vi "Mod_OFDM_Application.vi"(0 "Configure  Modulators Pool":bool, 1 "Configure OFDM Symbol":bool, 2 "Configure OFDM Frame":bool, 3 "Configure Pulse Shaping":bool, 4 "Write Configuration":bool, 5 "error in (no error)":errorcluster, 6 "Configure Data Pool":bool, 7 "Generate Waveform":bool, 8 "Read From File":bool, 9 "EXIT":bool) -> (12 "FFT Spectrum":cluster{dbl, dbl, dbl[]}(graph)={-798437.4999999999, 1562.4999999999998, [-inf, -inf, -inf, -inf, -inf, -inf, -inf, -inf, -inf, -inf, -inf, -inf, -inf, -inf, -inf, -inf, -inf, -inf, -inf, -inf, -inf, -inf, -inf, -inf, -inf, -inf, -inf, -inf, -inf, -inf, -inf, -inf, -inf, -inf, -inf, -inf, -inf, -inf, -inf, -inf, -inf, -inf, -inf, -inf, -inf, -inf, -inf, -inf, -inf, -inf, -inf, -inf, -inf, -inf, -inf, -inf, -inf, -inf, -inf, -inf, -inf, -inf, -inf, -inf, -inf, -inf, -inf, -inf, -inf, -inf, -inf, -inf, -inf, -inf, -inf, -inf, -inf, -inf, -inf, -inf, -inf, -inf, -inf, -inf, -inf, -inf, -inf, -inf, -inf, -inf, -inf, -inf, -inf, -inf, -inf, -inf, -inf, -inf, -inf, -inf, -inf, -inf, -inf, -inf, -inf, -inf, -inf, -inf, -inf, -inf, -inf, -inf, -inf, -inf, -inf, -inf, -inf, -inf, -inf, -inf, -inf, -inf, -inf, -inf, -inf, -inf, -inf, -inf, -inf, -inf, -inf, -inf, -inf, -inf, -inf, -inf, -inf, -inf, -inf, -inf, -inf, -inf, -inf, -inf, -inf, -inf, -inf, -inf, -inf, -inf, -inf, -inf, -inf, -inf, -inf, -inf, -inf, -inf, -inf, -inf, -inf, -inf, -inf, -inf, -inf, -inf, -inf, -inf, -inf, -inf, -inf, -inf, -inf, -inf, -inf, -inf, -inf, -inf, -inf, -inf, -inf, -inf, -inf, -inf, -inf, -inf, -inf, -inf, -inf, -inf, -inf, -inf, -inf, -inf, -inf, -inf, -inf, -inf, -inf, -inf, -inf, -inf, -inf, -inf, -inf, -inf, -inf, -inf, -inf, -inf, -inf, -inf, -inf, -inf, -inf, -inf, -inf, -inf, -inf, -inf, -inf, -inf, -inf, -inf, -inf, -inf, -inf, -inf, -inf, -inf, -inf, -inf, -inf, -inf, -inf, -inf, -inf, -inf, -inf, -inf, -inf, -inf, -inf, -inf, -inf, -inf, -inf, -inf, -inf, -inf, -inf, -inf, -inf, -inf, -inf, -inf, -inf, -inf, -inf, -inf, -inf, -inf, -inf, -inf, -inf, -inf, -inf, -inf, -inf, -inf, -inf, -inf, -inf, -inf, -inf, -inf, -inf, -inf, -inf, -inf, -inf, -inf, -inf, -inf, -inf, -inf, -inf, -inf, -inf, -inf, -inf, -inf, -inf, -inf, -inf, -inf, -inf, -inf, -inf, -inf, -inf, -inf, -inf, -inf, -inf, -inf, -inf, -inf, -inf, -inf, -inf, -inf, -inf, -inf, -inf, -inf, -inf, -inf, -inf, -inf, -inf, -inf, -inf, -inf, -inf, -inf, -inf, -inf, -inf, -inf, -inf, -inf, -inf, -inf, -inf, -inf, -inf, -inf, -inf, -inf, -inf, -inf, -inf, -inf, -inf, -inf, -inf, -inf, -inf, -inf, -inf, -inf, -inf, -inf, -inf, -inf, -inf, -inf, -inf, -inf, -inf, -inf, -inf, -inf, -inf, -inf, -inf, -inf, -inf, -inf, -inf, -inf, -inf, -inf, -inf, -inf, -inf, -inf, -inf, -inf, -inf, -inf, -inf, -inf, -inf, -inf, -inf, -inf, -inf, -inf, -inf, -inf, -inf, -inf, -inf, -inf, -inf, -inf, -inf, -inf, -inf, -inf, -inf, -inf, -inf, -inf, -inf, -inf, -inf, -inf, -inf, -inf, -inf, -inf, -inf, -inf, -inf, -inf, -inf, -inf, -inf, -inf, -inf, -inf, -inf, -inf, -inf, -inf, -inf, -inf, -inf, -inf, -inf, -inf, -inf, -inf, -inf, -inf, -inf, -inf, -inf, -inf, -inf, -inf, -inf, -inf, -inf, -inf, -inf, -inf, -inf, -inf, -inf, -inf, -inf, -inf, -inf, -inf, -inf, -inf, -inf, -inf, -inf, -inf, -inf, -inf, -inf, -inf, -inf, -inf, -inf, -inf, -inf, -inf, -inf, -inf, -inf, -inf, -inf, -inf, -inf, -inf, -inf, -inf, -inf, -inf, -inf, -inf, -inf, -inf, -inf, -inf, -inf, -inf, -inf, -inf, -inf, -inf, -inf, -inf, -inf, -inf, -inf, -inf, -inf, -inf, -inf, -inf, -inf, -inf, -inf, -inf, -inf, -inf, -inf, -inf, -inf, -inf, -inf, -inf, -inf, -inf, -inf, -inf, -inf, -inf, -inf, -inf, -inf, -inf, -inf, -inf, -inf, -inf, -inf, -inf, -inf, -inf, -inf, -inf, -inf, -inf, -inf, -inf, -inf, -inf, -inf, -inf, -inf, -inf, -inf, -inf, -inf, -inf, -inf, -inf, -inf, -inf, -inf, -inf, -inf, -inf, -inf, -inf, -inf, -inf, -inf, -inf, -inf, -inf, -inf, -inf, -inf, -inf, -inf, -inf, -inf, -inf, -inf, -inf, -inf, -inf, -inf, -inf, -inf, -inf, -inf, -inf, -inf, -inf, -inf, -inf, -inf, -inf, -inf, -inf, -inf, -inf, -inf, -inf, -inf, -inf, -inf, -inf, -inf, -inf, -inf, -inf, -inf, -inf, -inf, -inf, -inf, -inf, -inf, -inf, -inf, -inf, -inf, -inf, -inf, -inf, -inf, -inf, -inf, -inf, -inf, -inf, -inf, -inf, -inf, -inf, -inf, -inf, -inf, -inf, -inf, -inf, -inf, -inf, -inf, -inf, -inf, -inf, -inf, -inf, -inf, -inf, -inf, -inf, -inf, -inf, -inf, -inf, -inf, -inf, -inf, -inf, -inf, -inf, -inf, -inf, -inf, -inf, -inf, -inf, -inf, -inf, -inf, -inf, -inf, -inf, -inf, -inf, -inf, -inf, -inf, -inf, -inf, -inf, -inf, -inf, -inf, -inf, -inf, -inf, -inf, -inf, -inf, -inf, -inf, -inf, -inf, -inf, -inf, -inf, -inf, -inf, -inf, -inf, -inf, -inf, -inf, -inf, -inf, -inf, -inf, -inf, -inf, -inf, -inf, -inf, -inf, -inf, -inf, -inf, -inf, -inf, -inf, -inf, -inf, -inf, -inf, -inf, -inf, -inf, -inf, -inf, -inf, -inf, -inf, -inf, -inf, -inf, -inf, -inf, -inf, -inf, -inf, -inf, -inf, -inf, -inf, -inf, -inf, -inf, -inf, -inf, -inf, -inf, -inf, -inf, -inf, -inf, -inf, -inf, -inf, -inf, -inf, -inf, -inf, -inf, -inf, -inf, -inf, -inf, -inf, -inf, -inf, -inf, -inf, -inf, -inf, -inf, -inf, -inf, -inf, -inf, -inf, -inf, -inf, -inf, -inf, -inf, -inf, -inf, -inf, -inf, -inf, -inf, -inf, -inf, -inf, -inf, -inf, -inf, -inf, -inf, -inf, -inf, -inf, -inf, -inf, -inf, -inf, -inf, -inf, -inf, -inf, -inf, -inf, -inf, -inf, -inf, -inf, -inf, -inf, -inf, -inf, -inf, -inf, -inf, -inf, -inf, -inf, -inf, -inf, -inf, -inf, -inf, -inf, -inf, -inf, -inf, -inf, -inf, -inf, -inf, -inf, -inf, -inf, -inf, -inf, -inf, -inf, -inf, -inf, -inf, -inf, -inf, -inf, -inf, -inf, -inf, -inf, -inf, -inf, -inf, -inf, -inf, -inf, -inf, -inf, -inf, -inf, -inf, -inf, -inf, -inf, -inf, -inf, -inf, -inf, -inf, -inf, -inf, -inf, -inf, -inf, -inf, -inf, -inf, -inf, -inf, -inf, -inf, -inf, -inf, -inf, -inf, -inf, -inf, -inf, -inf, -inf, -inf, -inf, -inf, -inf, -inf, -inf, -inf, -inf, -inf, -inf, -inf, -inf, -inf, -inf, -inf, -inf, -inf, -inf, -inf, -inf, -inf, -inf, -inf, -inf, -inf, -inf, -inf, -inf, -inf, -inf, -inf, -inf, -inf, -inf, -inf, -inf, -inf, -inf, -inf, -inf, -inf, -inf, -inf, -inf, -inf, -inf, -inf, -inf, -inf, -inf, -inf, -inf, -inf, -inf, -inf, -inf, -inf, -inf, -inf, -inf, -inf, -inf, -inf, -inf, -inf, -inf, -inf, -inf, -inf, -inf, -inf, -inf, -inf, -inf, -inf, -inf, -inf, -inf, -inf, -inf, -inf, -inf, -inf, -inf, -inf, -inf, -inf, -inf, -inf, -inf, -inf, -inf, -inf, -inf, -inf, -inf, -inf, -inf, -inf, -inf, -inf, -inf, -inf, -inf, -inf, -inf, -inf, -inf, -inf, -inf, -inf, -inf, -inf, -inf, -inf, -inf, -inf, -inf, -inf, -inf, -inf, -inf, -inf, -inf, -inf, -inf, -inf, -inf, -inf]} caption="Baseband complex waveform", 14 "Complex Waveform":T1={"t0"=0.0, "dt"=1.0, "Y"=[]} {"Y" format="%.3f"; "dt" format="%^.2e"; "t0" format="%.4f"}, 15 "Results":T3, 16 "Status":T2={"Pool Size"=4, "Pool Size "=4, "OFDM Symbol?"=FALSE, "OFDM Frame?"=FALSE, "Sub Carriers"=64, "Cyclic Prefix"=16, "Tx Filter"=enum."Root Raised Cos"}, 19 "error out":errorcluster)   [LabVIEW 2010]
uses:
  <vilib>/addons/Modulation/Analog/controls/Complex Data Waveform.ctl
  Instance           8 28Saved   Mod_OFDM_Application .vi
  Instance           9 28Saved   Mod_OFDM_Application .vi
  Instance           7 28Saved   Mod_OFDM_Application .vi
panel:
  # "Step 0\nLoad Configuration\nfile   (optional)"
  # "Step 1\nConfigure/Examine\nPool of Data sources"
  # "Step 2\nConfigure/Examine\nPool of Modulators"
  # "Step 3\nConfigure/Examine\nOFDM Symbols"
  # "Step 4\nConfigure/Examine\nOFDM Frame"
  # "Step 5\nConfigure/Examine\nPulse Shaping"
  # "Step 6\nStore Configuration\nfile  (optional)"
  # "Step 7\nGenerate/Store\nWaveform"
  # "Step 8\nExit Application"
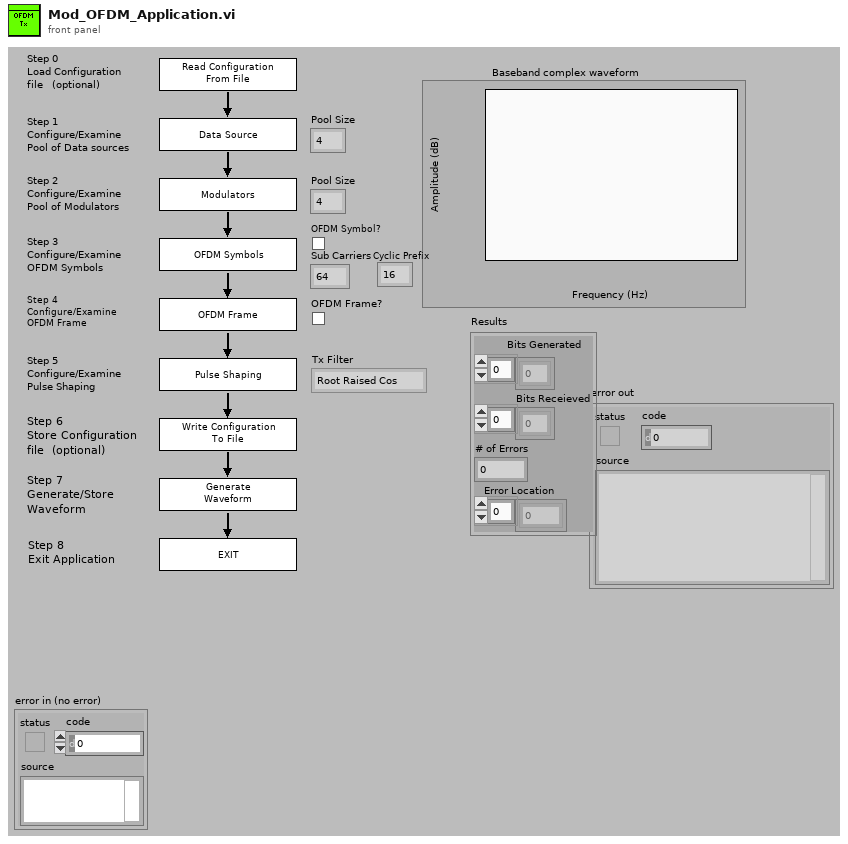
[diagram p1: front panel]
types:
  T1 = typedef "Complex Data Waveform.ctl" = cluster{"t0":dbl, "dt":dbl, "Y":cdb[]}
  T2 = cluster{"Pool Size":i32, "Pool Size ":i32, "OFDM Symbol?":bool, "OFDM Frame?":bool, "Sub Carriers":i32, "Cyclic Prefix":i32, "Tx Filter":enum16{"none", "Raised Cosine", "Root Raised Cos"}}
  T3 = cluster{"Bits Generated":i8[], "Bits Receieved":i8[], "# of Errors":i32, "Error Location":i32[]}
  T4 = cluster{"Pool Size":i32, "Pool Size":i32, "OFDM Symbol?":bool, "OFDM Frame?":bool, "Sub Carriers":i32, "Cyclic Prefix":i32, "TX Filter":enum16{"none", "Raised Cosine", "Root Raised Cos"}}
  T5 = cluster{"Phase Continous \nWaveform":bool, "Store Waveform\nTo a File":bool, "Generate Waveform":bool, "Store Waveform + \nConfiguration To Files":bool}
  T6 = typedef "Parameters per Ofdm Symbol.ctl" = cluster{"Length Of Cylic Prefix":i32, "# of Sub Carrier":i32, "Sub Carrier":bool[], "Data Source":cluster{"Data Source":u16, "Data Source":cluster{"mode (PN)":enum16{"PN", "pattern", "user"}, "PN sequence order (9)":i32, "Invert Output Bits":enum16{"No", "Yes"}, "Register Initial State":u32, "User base bit pattern":i8[], "base bit pattern (00001111)":enum16{"0", "1", "01", "0011", "00001111"}, "Reset to Initial State":enum16{"Every OFDM Frame", "Every OFDM Symbol", "Every Sub Carrier"}}}[], "Modulator Source":cluster{"Type of Modulation":enum16{"PSK", "QAM"}, "PSK":cluster{"differential PSK":enum16{"disable", "enable"}, "PSK type":u16}, "M-PSK/M-QAM":i32, "Bits per symbol":i32, "Modulator":u16}[], "Symbol Name":string}[]
  T7 = typedef "Configure Pulse Shaping.ctl" = cluster{"System Filter":cluster{"TX Filter":enum16{"none", "Raised Cosine", "Root Raised Cos"}, "Alpha":dbl, "filter length":i32}, "Modulation system parameters":cluster{"samples per symbol (16)":u32}, "symbol rate (Hz)":dbl}
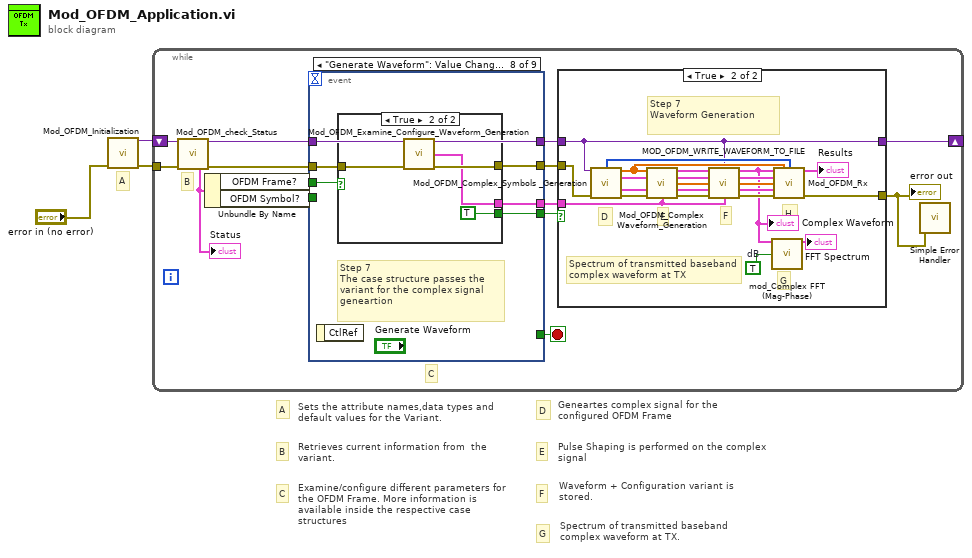
[diagram p0: block diagram]
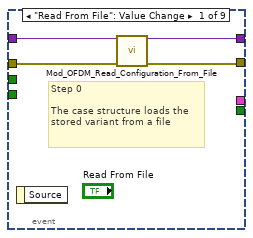
[diagram p3: hidden frame]
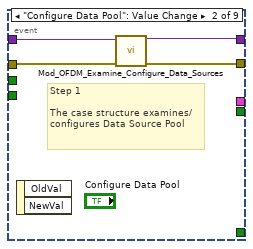
[diagram p4: hidden frame]
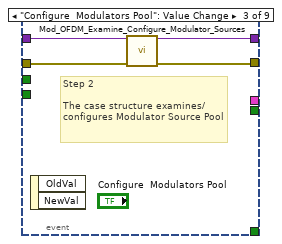
[diagram p5: hidden frame]
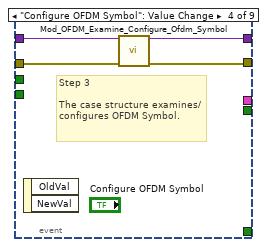
[diagram p6: hidden frame]
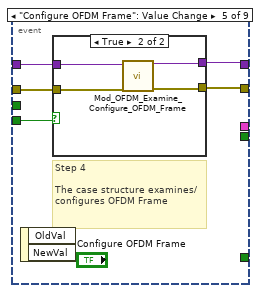
[diagram p7: hidden frame]
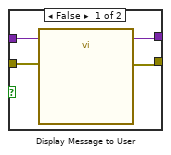
[diagram p8: hidden frame]
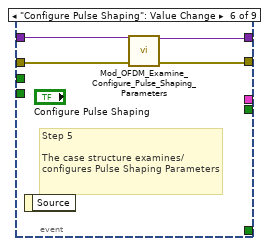
[diagram p9: hidden frame]
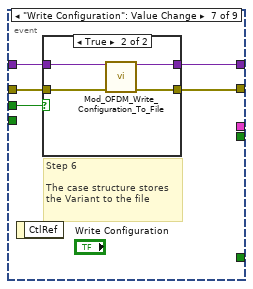
[diagram p10: hidden frame]
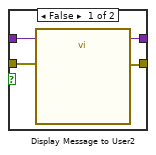
[diagram p11: hidden frame]
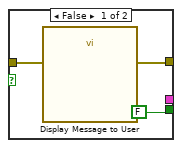
[diagram p12: hidden frame]
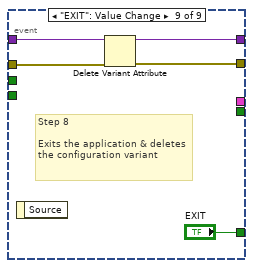
[diagram p13: hidden frame]
diagram:
  # "Waveform + Configuration variant is stored."
  # "G"
  # "Examine/configure different parameters for the OFDM Frame. More information is available inside the respective case structures"
  # "Spectrum of transmitted baseband\ncomplex waveform at TX."
  # "Pulse Shaping is performed on the complex signal"
  # "Geneartes complex signal for the configured OFDM Frame"
  # "Retrieves current information from  the variant."
  # "Sets the attribute names,data types and default values for the Variant."
  # "F"
  # "E"
  # "D"
  # "A"
  # "C"
  # "B"
  # "A"
  n1 = call "Mod_OFDM_Initialization.vi"("error in (no error)"="error in (no error)") -> ("Configuration out"=w2:variant, "error out"=w3:errorcluster)  [unwired: 13 in]
  n2 = while {
    shift-right: [w8] -> _
    shift-left: w2 -> [w17]
    tunnel: w3 -> [w15]
    stop <- w5 stop-if-true
    # "C"
    # "B"
    n3 = call "Mod_OFDM_check_Status.vi"("Configuration in"=w17, "error in"=w15) -> ("Configuration out"=w16:variant, "Status"=w7:T4, "error out"=w14:errorcluster)  [unwired: 11 in]
    "Status" <- w7
    n4 = Unbundle By Name(w7) -> ("OFDM Frame?"=w13:bool, "OFDM Symbol?"=w12:bool)
    n5 = event shown="[7] \"Generate Waveform\": Value Change" {
      selector: _ -> [_ _ _ _ _ _ _ _ _]
      dyn-events: _ -> [_ _ _ _ _ _ _ _ _]
      timeout: _ -> [_ _ _ _ _ _ _ _ _]
      tunnel: [w39 w45 w49 w53 w58 w69 w73 w88 w99] -> w10
      tunnel: w16 -> [w40 w46 w50 w54 w59 w70 w74 w88 w100]
      tunnel: [w41 w43 w47 w51 w56 w67 w71 w84 w97] -> w9
      tunnel: w14 -> [w42 w44 w48 w52 w57 w68 w72 w85 w98]
      tunnel: w13 -> [_ _ _ _ _ _ w75 w87 _]
      tunnel: w12 -> [_ _ _ _ w55 _ _ _ _]
      tunnel: [_ _ _ _ _ _ _ w86 _] -> w11
      tunnel: [_ _ _ _ _ _ _ _ "EXIT"] -> w5
      tunnel: [_ _ _ _ _ _ _ w83 _] -> w4
      event "Read From File": Value Change {
        # "Step 0\n\nThe case structure loads the stored variant from a file"
        n6 = event-data() -> ()  [unwired: 1 in, 1 out]
        n7 = call "Mod_OFDM_Read_Configuration_From_File.vi"("Configuration in"=w40, "error in"=w42) -> ("Configuration out"=w39:variant, "error out"=w41:errorcluster)  [unwired: 12 in]
      }
      event "Configure Data Pool": Value Change {
        # "Step 1\n\nThe case structure examines/configures Data Source Pool"
        n8 = event-data() -> ()  [unwired: 1 in, 2 out]
        n9 = call "Mod_OFDM_Examine_Configure_Data_Sources.vi"("Configuration in"=w46, "error in"=w44) -> ("Configuration out"=w45:variant, "error out"=w43:errorcluster)  [unwired: 12 in]
      }
      event "Configure  Modulators Pool": Value Change {
        # "Step 2\n\nThe case structure examines/configures Modulator Source Pool"
        n10 = event-data() -> ()  [unwired: 1 in, 2 out]
        n11 = call "Mod_OFDM_Examine_Configure_Modulator_Sources.vi"("Configuration in"=w50, "error in"=w48) -> ("Configuration out"=w49:variant, "error out"=w47:errorcluster)  [unwired: 12 in]
      }
      event "Configure OFDM Symbol": Value Change {
        # "Step 3\n\nThe case structure examines/configures OFDM Symbol."
        n12 = event-data() -> ()  [unwired: 1 in, 2 out]
        n13 = call "Mod_OFDM_Examine_Configure_Ofdm_Symbol.vi"("Configuration in"=w54, "error in"=w52) -> ("Configuration out"=w53:variant, "error out"=w51:errorcluster)  [unwired: 12 in]
      }
      event "Configure OFDM Frame": Value Change {
        # "Step 4\n\nThe case structure examines/configures OFDM Frame"
        n14 = event-data() -> ()  [unwired: 1 in, 2 out]
        n15 = case shown="True" w55 {
          tunnel: w59 -> [w62 w66]
          tunnel: [w62 w65] -> w58
          tunnel: w57 -> [w61 w64]
          tunnel: [w60 w63] -> w56
          frame False {
            n16 = call "Display Message to User"("error in (no error)"=w61) -> ("error out"=w60:errorcluster)  [unwired: 9 in, 1 out]
          }
          frame True {
            n17 = call "Mod_OFDM_Examine_Configure_OFDM_Frame.vi"("Configuration in"=w66, "error in"=w64) -> ("Configuration out"=w65:variant, "error out"=w63:errorcluster)  [unwired: 12 in]
          }
        }
      }
      event "Configure Pulse Shaping": Value Change {
        # "Step 5\n\nThe case structure examines/configures Pulse Shaping Parameters"
        n18 = event-data() -> ()  [unwired: 1 in, 1 out]
        n19 = call "Mod_OFDM_Examine_Configure_Pulse_Shaping_Parameters.vi"("Configuration in"=w70, "error in"=w68) -> ("Configuration out"=w69:variant, "error out"=w67:errorcluster)  [unwired: 12 in]
      }
      event "Write Configuration": Value Change {
        # "Step 6\n\nThe case structure stores the Variant to the file"
        n20 = event-data() -> ()  [unwired: 1 in, 1 out]
        n21 = case shown="True" w75 {
          tunnel: w74 -> [w78 w82]
          tunnel: [w78 w81] -> w73
          tunnel: w72 -> [w77 w80]
          tunnel: [w76 w79] -> w71
          frame False {
            n22 = call "Display Message to User2"("error in (no error)"=w77) -> ("error out"=w76:errorcluster)  [unwired: 9 in, 1 out]
          }
          frame True {
            n23 = call "Mod_OFDM_Write_Configuration_To_File.vi"("Configuration in"=w82, "error in"=w80) -> ("Configuration out"=w81:variant, "error out"=w79:errorcluster)  [unwired: 12 in]
          }
        }
      }
      event "Generate Waveform": Value Change {
        # "Step 7\nThe case structure passes the variant for the complex signal  geneartion"
        n24 = event-data() -> ()  [unwired: 1 in, 1 out]
        n25 = case shown="True" w87 {
          tunnel: [FALSE ("Generate Waveform") TRUE ("Generate Waveform")] -> w86
          tunnel: w85 -> [w91 w95]
          tunnel: [w90 w94] -> w84
          tunnel: [_ w92] -> w83
          frame False {
            n26 = call "Display Message to User"("error in (no error)"=w91) -> ("error out"=w90:errorcluster)  [unwired: 9 in, 1 out]
          }
          frame True {
            n27 = call "Mod_OFDM_Examine_Configure_Waveform_Generation.vi"("error in"=w95) -> ("Config_Waveform"=w92:T5, "error out"=w94:errorcluster)  [unwired: 13 in]
          }
        }
      }
      event "EXIT": Value Change {
        # "Step 8\n\nExits the application & deletes the configuration variant"
        n28 = event-data() -> ()  [unwired: 1 in, 1 out]
        n29 = Delete Variant Attribute(4:w98, 7:w100) -> (0:w97:errorcluster, 3:w99:variant)  [unwired: 1 in, 1 out]
      }
    }
    n30 = case shown="True" w11 {
      tunnel: w10 -> [w19 w20]
      tunnel: w9 -> [w18 w32]
      tunnel: [w19 w20] -> w8
      tunnel: [w18 w26] -> w6
      tunnel: w4 -> [_ w21]
      frame False {
      }
      frame True {
        w25 = TRUE  # dB
        # "Step 7\nWaveform Generation"
        # "H"
        # "Spectrum of transmitted baseband\ncomplex waveform at TX"
        # "G"
        # "F"
        # "E"
        # "D"
        n31 = call "Mod_OFDM_Complex_Symbols _Generation.vi"("Configuration in"=w20, "error in (no error)"=w32) -> ("Bits Generated"=w36:i8[], "Complex Symbols w/ Cyclic prefix"=w24:cdb[], "Parameters per Ofdm Symbol"=w35:T6, "Pulse Shaping Parameters"=w34:T7, "error out"=w33:errorcluster)  [unwired: 7 in, 2 out]
        n32 = call "Mod_OFDM_Complex Waveform_Generation.vi"("Complex Symbols \nw/ Cyclic prefix"=w24, "Parameters per Ofdm Symbol"=w35, "Pulse Shaping"=w34, "error in (no error)"=w33, "Config_Waveform"=w21) -> ("output complex waveform"=w23:T1, "Parameters per Ofdm Symbol"=w30:T6, "matched filter coefficients"=w28:dbl[], "Pulse Shaping"=w29:T7, "error out"=w31:errorcluster)  [unwired: 6 in]
        n33 = call "MOD_OFDM_WRITE_WAVEFORM_TO_FILE.VI"("Complex Waveform"=w23, "Configuration in"=w20, "error IO"=w31, "Config_Waveform"=w21) -> ("Complex Waveform"=w22:T1, "error out"=w27:errorcluster)  [unwired: 10 in]
        "Complex Waveform" <- w22
        n34 = call <vilib>:"mod_Complex FFT (Mag-Phase).vi"("Input Data Waveform"=w22, "dB (on/off)"=w25) -> ("Magnitude"=→"FFT Spectrum":cluster{"f0":dbl, "df":dbl, "Y":dbl[]})  [unwired: 12 in, 1 out]
        n35 = call "Mod_OFDM_Rx.vi"("input complex waveform"=w22, "Complex Symbols w/ Cyclic prefix"=w24, "BitsTransmitted"=w36, "Parameters per Ofdm Symbol"=w30, "matched filter coefficients"=w28, "Pulse Shaping"=w29, "error in (no error)"=w27) -> ("o/p"=→"Results":T3, "error out"=w26:errorcluster)  [unwired: 6 in, 1 out]
      }
    }
    "error out" <- w6
    n36 = call <vilib>:"Simple Error Handler.vi"("error in (no error)"=w6) -> ()  [unwired: 4 in, 5 out]
  }
